vi "Select Device Dialog.vi"(7 "Filter Type":T1=enum."Product Name", 8 "error in (no error)":errorcluster, 10 "Filter Names":string[](array[string]), 11 "Item Ref in":T2 format="%.0x") -> (0 "error out":errorcluster, 1 "Cancelled?":bool, 2 "Selected Alias":string, 3 "Item Ref out":T2=18446744073709551615 format="%.0x")   [LabVIEW 2018, in "NIVS Hardware Discovery.lvlib"]
uses:
  NIVS Hardware Discovery.lvlib
  <vilib>/NI Veristand/Custom Device API/Custom Device Item Ref.ctl
  _Types/Filter Type.ctl
  <vilib>/NI Veristand/Custom Device API/Custom Device API.lvlib
panel:
  in  "Cancel":bool
  in  "Use Selected":bool
  in  "Refresh":bool
  in  "Compatible Devices":u16(ring)
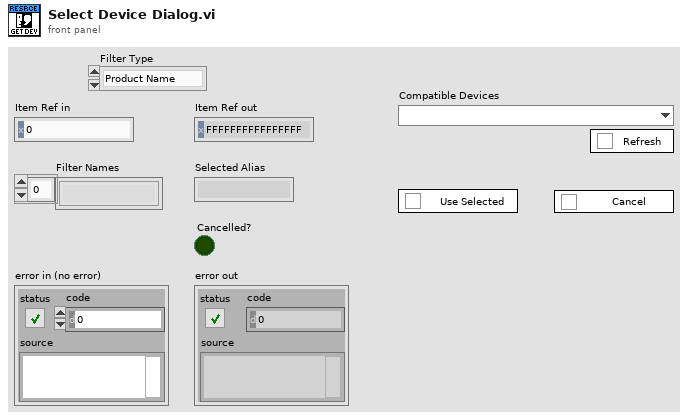
[diagram p1: front panel]
types:
  T1 = typedef "NIVS Hardware Discovery.lvlib/Filter Type.ctl" = enum16{"Device Category", "Product Name", "Ethernet", "XNET", "VISA", "FPGA", "EtherCAT Master", "DAQmx", "GPIB", "Serial"}
  T2 = typedef "Custom Device API.lvlib/Custom Device Item Ref.ctl" = u64
  T3 = enum32{"Invalid", "Standard", "Closed", "Hidden", "Minimized", "Maximized"}
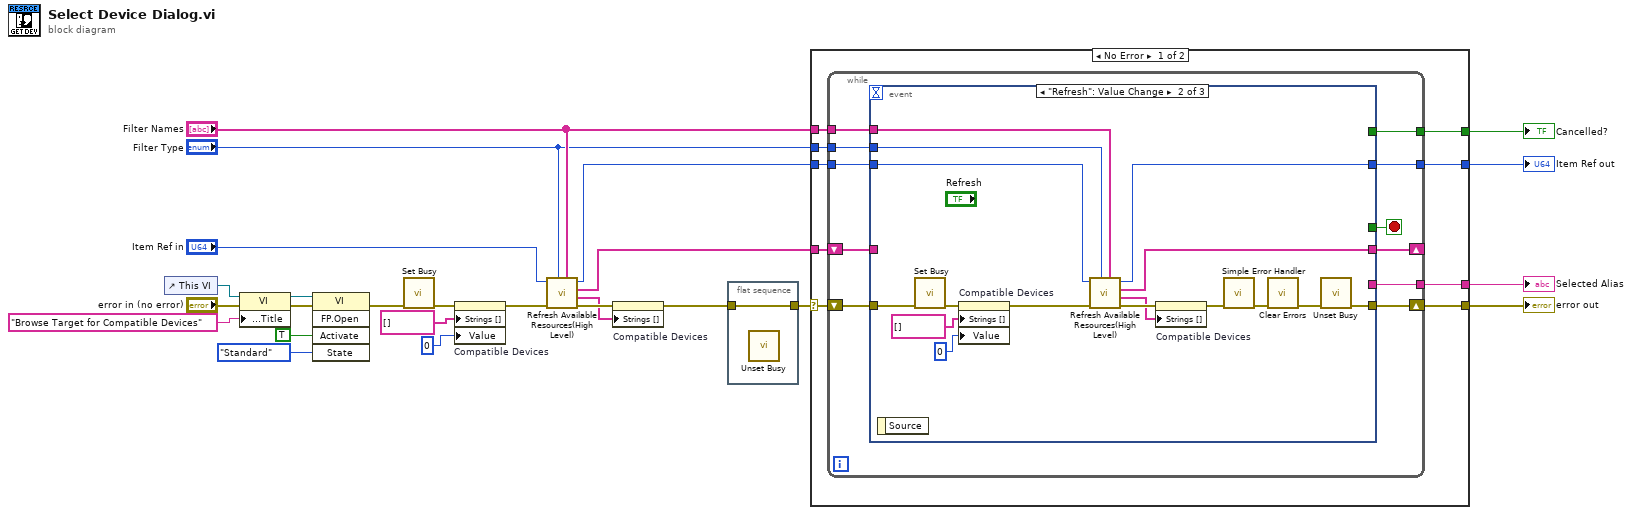
[diagram p0: block diagram]
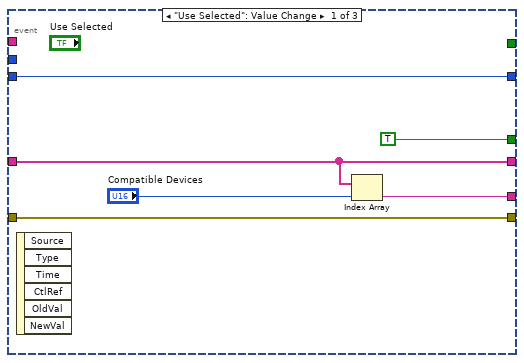
[diagram p2: hidden frame]
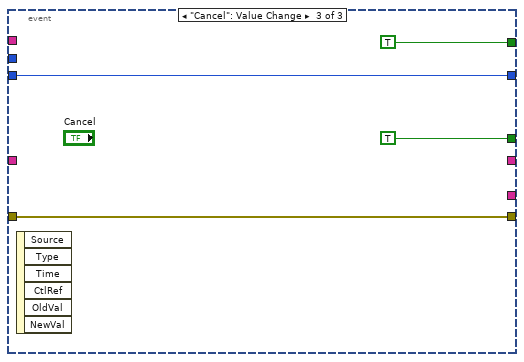
[diagram p3: hidden frame]
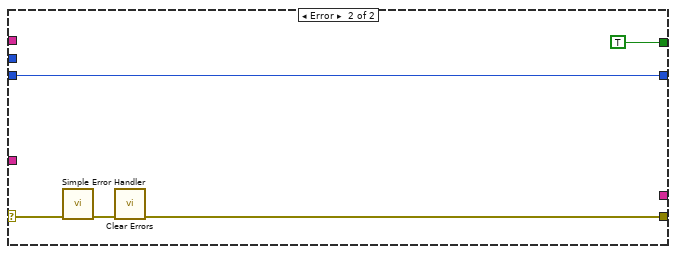
[diagram p4: hidden frame]
diagram:
  n1 = control-ref of="This VI"() -> (w17:refnum<vi>)
  n2 = property class="VI"(reference=w17, error in="error in (no error)", "Front Panel.Title"="Browse Target for Compatible Devices" ("Front Panel Window:Title")) -> (reference out=w15:refnum<vi>, error out=w14:errorcluster)
  n3 = invoke class="VI" method="FP.Open"(reference=w15, error in=w14, "Activate"=TRUE ("Activate?"), "State"=T3."Standard") -> (error out=w5:errorcluster)  [unwired: 1 in, 4 out]
  n4 = call <vilib>:"Set Busy.vi"("error in (no error)"=w5) -> ("error out"=w4:errorcluster)  [unwired: 9 in, 1 out]
  n5 = property on="Compatible Devices" class="Ring (strict)"(error in=w4, "Strings []"=string[] [], "Value"=0) -> (error out=w7:errorcluster)  [unwired: 1 in, 1 out]
  n6 = call "Refresh Available Resources(High Level).vi"("Filter Names"="Filter Names", "Filter Type"="Filter Type", "error in (no error)"=w7, "Section Ref in"="Item Ref in") -> ("error out"=w10:errorcluster, "Name and Alias"=w8:string[], "Aliases"=w9:string[], "Section Ref out"=w11:T2)  [unwired: 4 in]
  n7 = property on="Compatible Devices" class="Ring (strict)"(error in=w10, "Strings []"=w8) -> (error out=w2:errorcluster)  [unwired: 1 in, 1 out]
  n8 = flat-sequence {
    tunnel: [w26] -> w3
    tunnel: w2 -> [w26]
    frame #0 {
      n9 = call <vilib>:"Unset Busy.vi"() -> ()  [unwired: 11 in, 1 out]
    }
  }
  n10 = case shown="No Error" w3 {
    selector: w3 -> [w27 w77]
    tunnel: [w35 w74] -> w24
    tunnel: [w34 _] -> w23
    tunnel: "Filter Names" -> [w33 _]
    tunnel: [w32 TRUE] -> w21
    tunnel: [w31 w75] -> w18
    tunnel: "Filter Type" -> [w30 _]
    tunnel: w11 -> [w29 w74]
    tunnel: w9 -> [w28 _]
    frame No Error {
      n11 = while {
        shift-right: [w42] -> w31
        shift-left: w27 -> [w43]
        tunnel: [w45] -> w34
        tunnel: w29 -> [w41]
        shift-right: [w39] -> _
        shift-left: w28 -> [w46]
        tunnel: w33 -> [w40]
        tunnel: [w38] -> w32
        tunnel: [w37] -> w35
        tunnel: w30 -> [w36]
        stop <- w44 stop-if-true
        n12 = event shown="[1] \"Refresh\": Value Change" {
          selector: _ -> [_ _ _]
          dyn-events: _ -> [_ _ _]
          timeout: _ -> [_ _ _]
          tunnel: w46 -> [w48 _ _]
          tunnel: [w51 _ _] -> w45
          tunnel: [TRUE _ TRUE] -> w44
          tunnel: w43 -> [w49 w57 w69]
          tunnel: [w49 w54 w69] -> w42
          tunnel: w41 -> [w47 w68 w70]
          tunnel: w40 -> [_ w64 _]
          tunnel: [w48 w63 _] -> w39
          tunnel: [_ _ TRUE] -> w38
          tunnel: [w47 w67 w70] -> w37
          tunnel: w36 -> [_ w65 _]
          event "Use Selected": Value Change {
            n13 = event-data() -> ()  [unwired: 1 in, 6 out]
            n14 = Index Array(array=w48, index="Compatible Devices") -> (element=w51:string)
          }
          event "Refresh": Value Change {
            n15 = event-data() -> ()  [unwired: 1 in, 1 out]
            n16 = call <vilib>:"Set Busy.vi"("error in (no error)"=w57) -> ("error out"=w56:errorcluster)  [unwired: 9 in, 1 out]
            n17 = property on="Compatible Devices" class="Ring (strict)"(error in=w56, "Strings []"=string[] [], "Value"=0) -> (error out=w59:errorcluster)  [unwired: 1 in, 1 out]
            n18 = call "Refresh Available Resources(High Level).vi"("Filter Names"=w64, "Filter Type"=w65, "error in (no error)"=w59, "Section Ref in"=w68) -> ("error out"=w66:errorcluster, "Name and Alias"=w62:string[], "Aliases"=w63:string[], "Section Ref out"=w67:T2)  [unwired: 4 in]
            n19 = property on="Compatible Devices" class="Ring (strict)"(error in=w66, "Strings []"=w62) -> (error out=w60:errorcluster)  [unwired: 1 in, 1 out]
            n20 = call <vilib>:"Simple Error Handler.vi"("error in (no error)"=w60) -> ("error out"=w61:errorcluster)  [unwired: 4 in, 4 out]
            n21 = call <vilib>:"Clear Errors.vi"("error in (no error)"=w61) -> ("error out"=w55:errorcluster)  [unwired: 5 in, 1 out]
            n22 = call <vilib>:"Unset Busy.vi"("error in (no error)"=w55) -> ("error out"=w54:errorcluster)  [unwired: 10 in]
          }
          event "Cancel": Value Change {
            n23 = event-data() -> ()  [unwired: 1 in, 6 out]
          }
        }
      }
    }
    frame Error {
      n24 = call <vilib>:"Simple Error Handler.vi"("error in (no error)"=w77) -> ("error out"=w76:errorcluster)  [unwired: 4 in, 4 out]
      n25 = call <vilib>:"Clear Errors.vi"("error in (no error)"=w76) -> ("error out"=w75:errorcluster)  [unwired: 5 in, 1 out]
    }
  }
  "error out" <- w18
  "Item Ref out" <- w24
  "Selected Alias" <- w23
  "Cancelled?" <- w21
